vi "addTab.vi"(6 "label":string, 8 "Error In":errorcluster, 9 "icon":refnum<class "QIcon.lvclass">, 10 "widget":refnum<class "QWidget.lvclass">, 11 "QTabWidget In":refnum<class "QTabWidget.lvclass">) -> (0 "Error Out":errorcluster, 2 "Value":i32, 3 "QTabWidget Out":refnum<class "QTabWidget.lvclass">)   [LabVIEW 2014, in "QTabWidget.lvclass"]
doc: "LabVIEW-specific documentation is not yet available. See <b>http://doc.qt.io/qt-5/QTabWidget.html#addTab</b>"
uses:
  QTabWidget.lvclass
  QWidget/QWidget.lvclass
  Qt GUI/QIcon/QIcon.lvclass
  LQ Core/LQIdentity/LQIdentity.lvclass/LQIdentity.ctl
  LQ Core/LQSerialData/LQSerialData.lvclass/LQSerialData.ctl
  LQ Core/LQ Core.lvlib
  LQ Core/LQIdentity/LQIdentity.lvclass
  LQ Core/LQSerialData/LQSerialData.lvclass
panel:
  # "Copyright (c) 2016 Sze Howe Koh\n\nThis Source Code Form is subject to the terms of the Mozilla Public\nLicense, v. 2.0. If a copy of the MPL was not distributed with this\nfile, You can obtain one at http://mozilla.org/MPL/2.0/."
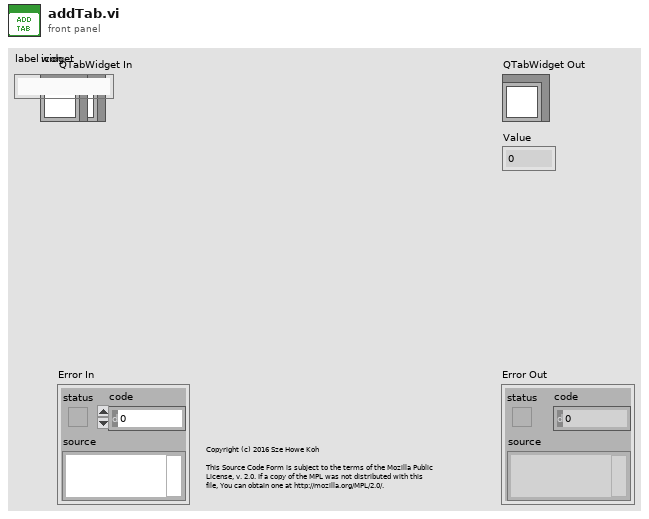
[diagram p1: front panel]
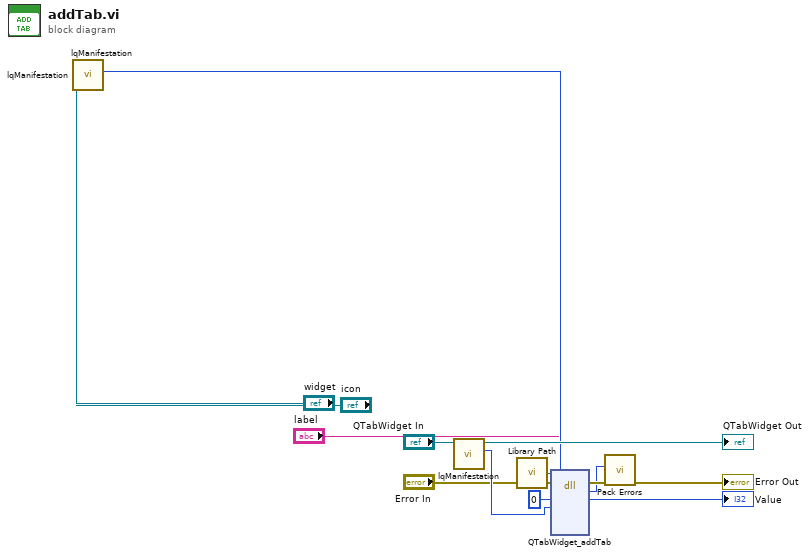
[diagram p0: block diagram]
diagram:
  n1 = call "lqManifestation.vi"("LQSerialData in"="icon") -> ("Manifestation"=w2:string)  [unwired: 9 in, 1 out]
  n2 = call "lqManifestation.vi"("LQIdentity in"="widget") -> ("Manifestation"=w4:u64)  [unwired: 9 in, 1 out]
  n3 = call "lqManifestation.vi"("LQIdentity in"="QTabWidget In") -> ("Manifestation"=w10:u64, "LQIdentity out"=→"QTabWidget Out":refnum<class "QTabWidget.lvclass">)  [unwired: 9 in]
  n4 = call "Library Path.vi"() -> ("Library Path"=w11:path)
  n5 = dll-call lib="?" fn="QTabWidget_addTab"(path in=w11, error in="Error In", "_retVal"=0 ("retVal"), "_instance"=w10, "widget"=w4, "icon"=w2, "label"="label") -> (error out=w8:errorcluster, w6:i32, "_retVal"=→"Value":i32)  [unwired: 5 in, 1 out]
  n6 = call "Pack Errors.vi"("Error In"=w8, "Error Code"=w6) -> ("Error Out"=→"Error Out":errorcluster)  [unwired: 9 in]
